vi "Update RPC Client Method Controls.vi"(5 "Server class in":refnum<vi>, 7 "RPC Method Parameters":T1[](array[typedef]), 8 "error in (no error)":errorcluster, 10 "RPC Method Name":string, 11 "VI in":refnum<vi>) -> (0 "error out":errorcluster, 3 "VI out":refnum<vi>)   [LabVIEW 2019, in "gRPC Scripting Tools.lvlib"]
uses:
  gRPC Scripting Tools.lvlib
  TypeDefs/RPC Method Parameters.ctl
  <vilib>/Utility/traverseref.llb/TRef TravTarget.ctl
  63320222-a0c5-46f2-a668-ff10f55be25f.vi
  108da764-e401-4abd-a40a-091b83fc4494.vi
  <vilib>/Comparison/Equal/Equal Functor/Equal Functor.lvclass
  <vilib>/Utility/traverseref.llb/VI Scripting - Traverse.lvlib
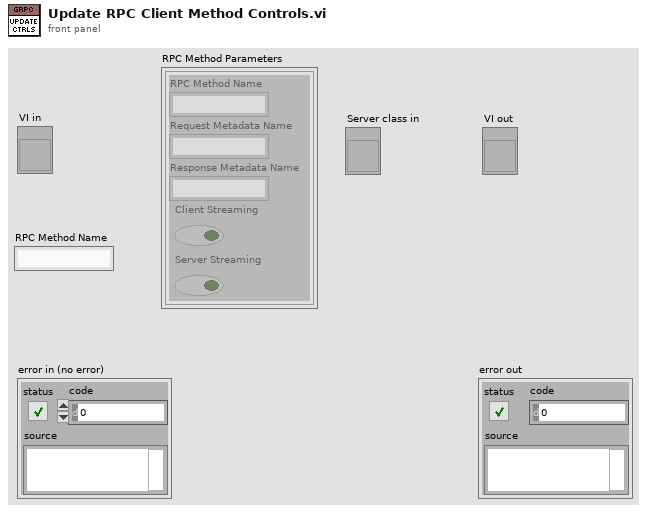
[diagram p1: front panel]
types:
  T1 = typedef "gRPC Scripting Tools.lvlib/RPC Method Parameters.ctl" = cluster{"RPC Method Name":string, "Request Metadata Name":string, "Response Metadata Name":string, "Client Streaming":bool, "Server Streaming":bool}
  T2 = typedef "TRef TravTarget.ctl" = enum16{"FP", "BD", "Other"}
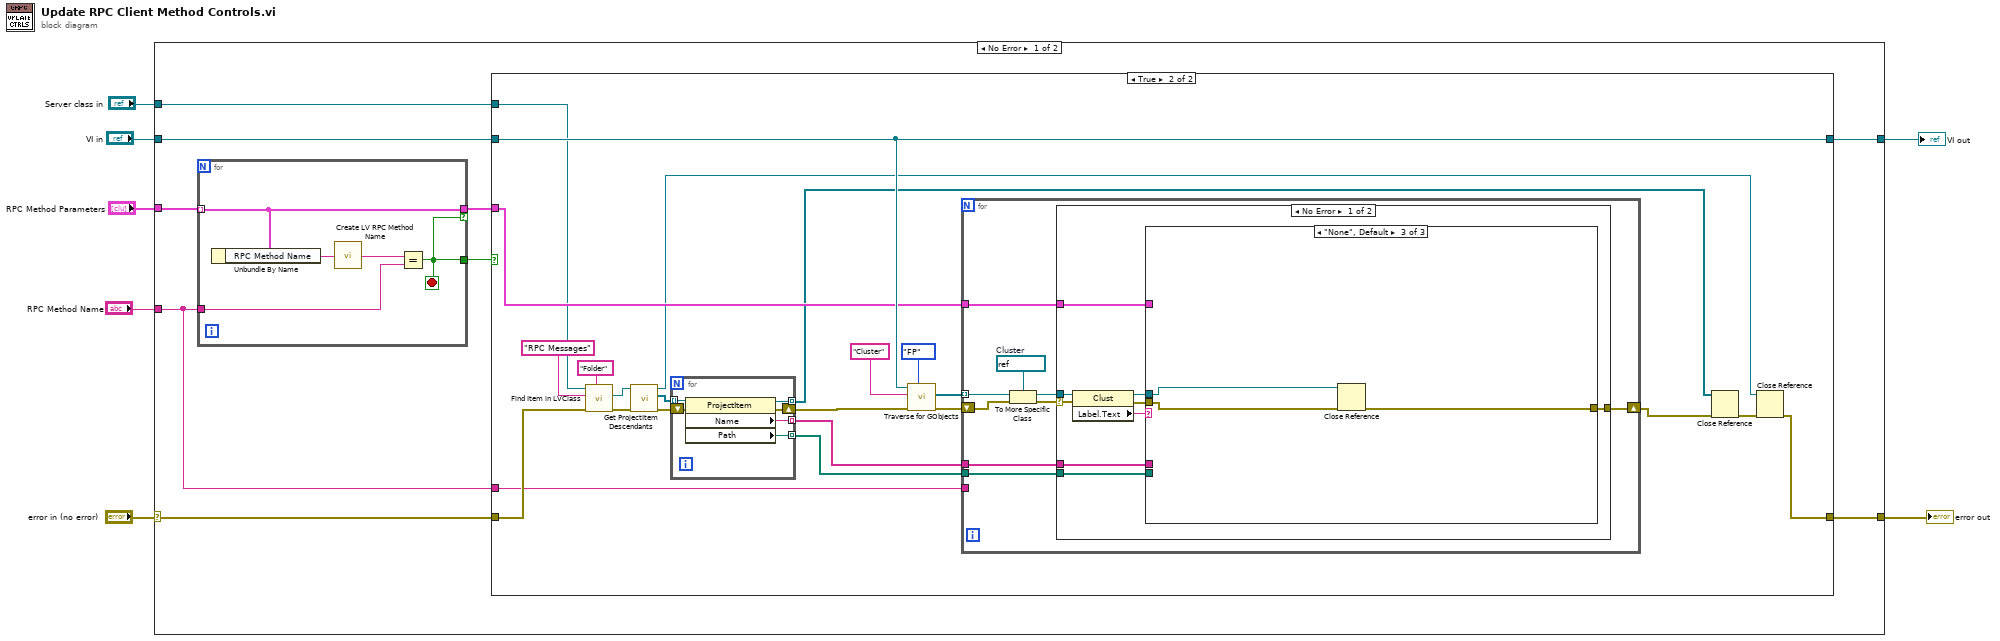
[diagram p0: block diagram]
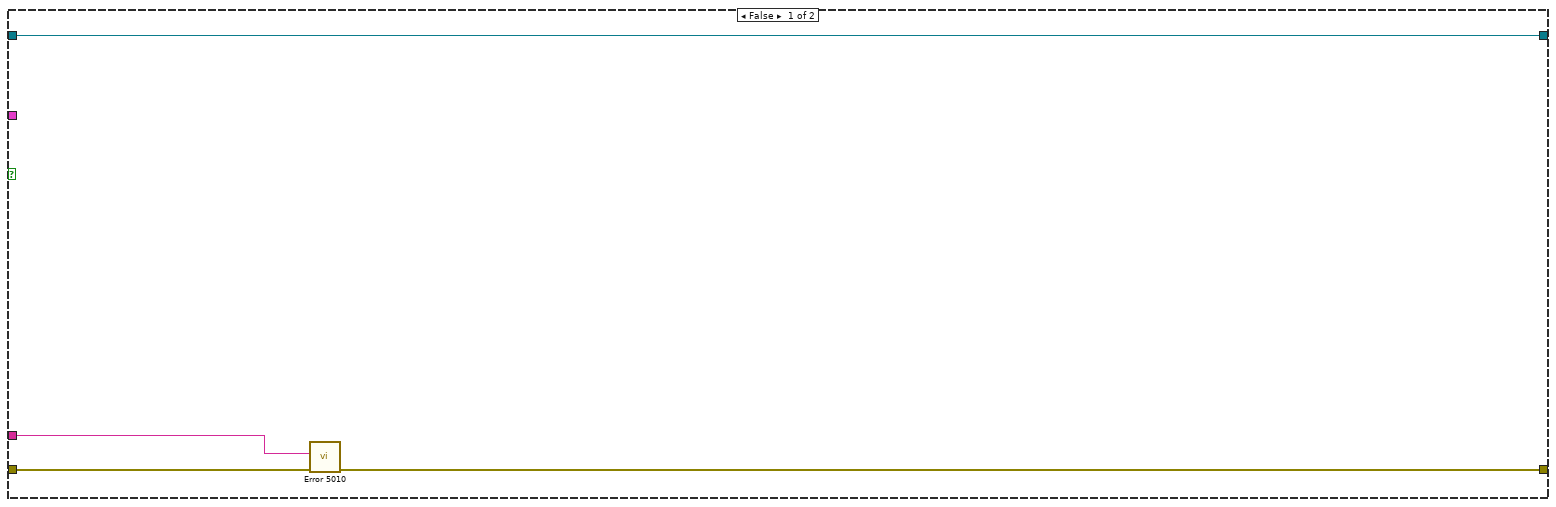
[diagram p2: hidden frame]
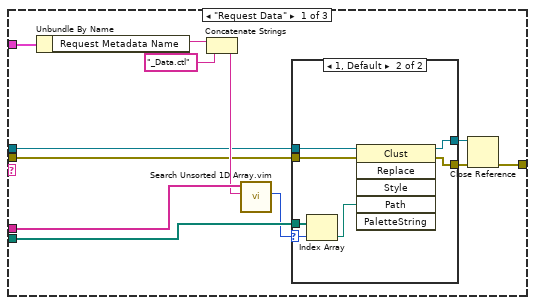
[diagram p3: hidden frame]
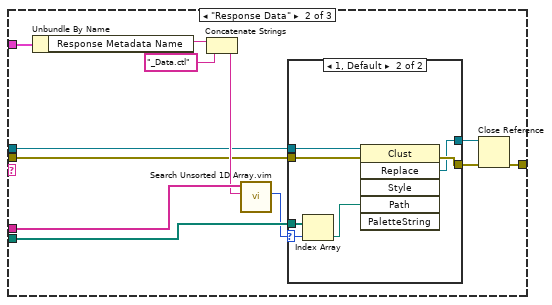
[diagram p5: hidden frame]
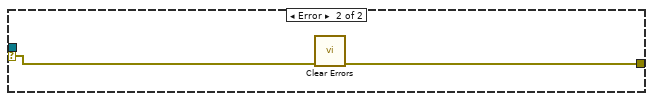
[diagram p7: hidden frame]
diagram:
  n1 = case shown="No Error" "error in (no error)" {
    selector: "error in (no error)" -> [w11 w121]
    tunnel: [w16 w121] -> w7
    tunnel: "VI in" -> [w15 w120]
    tunnel: "RPC Method Parameters" -> [w14 _]
    tunnel: "RPC Method Name" -> [w9 _]
    tunnel: [w10 w120] -> w2
    tunnel: "Server class in" -> [w8 _]
    frame No Error {
      n2 = for {
        tunnel: w14 -> [w118] mode=indexing
        tunnel: w9 -> [w119]
        tunnel: [w118] -> w12 if=w117
        tunnel: [w117] -> w13
        stop <- w117 stop-if-true
        n3 = Unbundle By Name(w118) -> ("RPC Method Name"=w116:string)
        n4 = call "Create LV RPC Method Name.vi"("Proto Parser RPC Method Name in"=w116) -> ("LV RPC Method Name out"=w115:string)
        n5 = Equal?(x=w115, y=w119) -> (x = y?=w117:bool)
      }
      n6 = case shown="True" w13 {
        tunnel: [w17 w22] -> w16
        tunnel: w11 -> [w19 w43]
        tunnel: w15 -> [w20 w40]
        tunnel: w12 -> [_ w36]
        tunnel: [w20 w40] -> w10
        tunnel: w9 -> [w18 w37]
        tunnel: w8 -> [_ w28]
        frame False {
          n7 = call "Error 5010.vi"("error in (no error)"=w19, "RPC Method Name"=w18) -> ("error out"=w17:errorcluster)  [unwired: 9 in]
        }
        frame True {
          n8 = call "Find Item in LVClass.vi"("Item Type"="Folder", "error in (no error)"=w43, "Item Name"="RPC Messages", "Class Item in"=w28) -> ("error out"=w34:errorcluster, "Project Item (Class Item)"=w33:refnum<vi>)  [unwired: 4 in, 2 out]
          n9 = call "Get ProjectItem Descendants.vi"("error in (no error)"=w34, "ProjectItem in"=w33) -> ("error out"=w30:errorcluster, "All Descendents"=w35:refnum<vi>[], "ProjectItem out"=w27:refnum<vi>)  [unwired: 7 in]
          n10 = for {
            tunnel: w35 -> [w49] mode=indexing
            tunnel: [w48] -> w26 mode=indexing
            tunnel: [w47] -> w25 mode=indexing
            shift-right: [w45] -> w29
            shift-left: w30 -> [w46]
            tunnel: [w44] -> w24 mode=indexing
            n11 = property class="ProjectItem"(reference=w49, error in=w46) -> (reference out=w47:refnum<vi>, error out=w45:errorcluster, "Name"=w48:string, "Path"=w44:path)
          }
          n12 = call <vilib>:"Traverse for GObjects.vi"("Traverse Target"=TRef_TravTarget."FP", "error in (no error)"=w29, "Class Name"="Cluster", "VI Refnum"=w40) -> ("error out"=w39:errorcluster, "References"=w38:refnum<vi>[])  [unwired: 4 in, 2 out]
          n13 = for {
            tunnel: w38 -> [w57] mode=indexing
            shift-right: [w53] -> w21
            shift-left: w39 -> [w56]
            tunnel: w37 -> [_]
            tunnel: w36 -> [w52]
            tunnel: w26 -> [w51]
            tunnel: w24 -> [w50]
            w58 = refnum<vi> refnum  # Cluster
            n14 = To More Specific Class(target class=w58, reference=w57, error in=w56) -> (specific class reference=w55:refnum<vi>, error out=w54:errorcluster)
            n15 = case shown="No Error" w54 {
              selector: w54 -> [w66 w114]
              tunnel: w55 -> [w67 _]
              tunnel: [w62 w113] -> w53
              tunnel: w52 -> [w61 _]
              tunnel: w51 -> [w60 _]
              tunnel: w50 -> [w59 _]
              frame No Error {
                n16 = property class="Clust"(reference=w67, error in=w66) -> (reference out=w64:refnum<vi>, error out=w63:errorcluster, "Label.Text"=w65:string)
                n17 = case shown="\"None\", Default" w65 {
                  tunnel: w64 -> [w72 w93 w110]
                  tunnel: w63 -> [w71 w92 w112]
                  tunnel: [w69 w89 w111] -> w62
                  tunnel: w61 -> [w79 w100 _]
                  tunnel: w60 -> [w76 w97 _]
                  tunnel: w59 -> [w74 w95 _]
                  frame "Request Data" {
                    n18 = Unbundle By Name(w79) -> ("Request Metadata Name"=w78:string)
                    n19 = Concatenate Strings(w78, "_Data.ctl" ("string")) -> (w75:string)
                    n20 = call "Search Unsorted 1D Array.vim"("element"=w75, "unsorted 1D array"=w76) -> ("index of element"=w73:i32)  [unwired: 9 in]
                    n21 = case shown="1, Default" w73 {
                      selector: w73 -> [_ w87]
                      tunnel: w74 -> [_ w88]
                      tunnel: w72 -> [w80 w86]
                      tunnel: w71 -> [w81 w85]
                      tunnel: [w81 w83] -> w70
                      tunnel: [w80 w82] -> w68
                      frame -1 {
                      }
                      frame 1, Default {
                        n22 = Index Array(array=w88, index=w87) -> (element=w84:path)
                        n23 = invoke class="Clust" method="Replace"(reference=w86, error in=w85, "Path"=w84) -> (reference out=w82:refnum<vi>, error out=w83:errorcluster)  [unwired: 3 in, 4 out]
                      }
                    }
                    n24 = Close Reference(reference=w68, error in (no error)=w70) -> (error out=w69:errorcluster)
                  }
                  frame "Response Data" {
                    n25 = Unbundle By Name(w100) -> ("Response Metadata Name"=w99:string)
                    n26 = Concatenate Strings(w99, "_Data.ctl" ("string")) -> (w96:string)
                    n27 = call "Search Unsorted 1D Array.vim"("element"=w96, "unsorted 1D array"=w97) -> ("index of element"=w94:i32)  [unwired: 9 in]
                    n28 = case shown="1, Default" w94 {
                      selector: w94 -> [_ w108]
                      tunnel: w95 -> [_ w109]
                      tunnel: w93 -> [w101 w107]
                      tunnel: [w101 w103] -> w90
                      tunnel: w92 -> [w102 w106]
                      tunnel: [w102 w105] -> w91
                      frame -1 {
                      }
                      frame 1, Default {
                        n29 = Index Array(array=w109, index=w108) -> (element=w104:path)
                        n30 = invoke class="Clust" method="Replace"(reference=w107, error in=w106, "Path"=w104) -> (error out=w105:errorcluster, "Replace"=w103:refnum<vi>)  [unwired: 3 in, 4 out]
                      }
                    }
                    n31 = Close Reference(reference=w90, error in (no error)=w91) -> (error out=w89:errorcluster)
                  }
                  frame "None", Default {
                    n32 = Close Reference(reference=w110, error in (no error)=w112) -> (error out=w111:errorcluster)
                  }
                }
              }
              frame Error {
                n33 = call <vilib>:"Clear Errors.vi"("error in (no error)"=w114) -> ("error out"=w113:errorcluster)  [unwired: 5 in, 1 out]
              }
            }
          }
          n34 = Close Reference(reference=w25, error in (no error)=w21) -> (error out=w23:errorcluster)
          n35 = Close Reference(reference=w27, error in (no error)=w23) -> (error out=w22:errorcluster)
        }
      }
    }
    frame Error {
    }
  }
  "error out" <- w7
  "VI out" <- w2
